vi "CMN_toMdMgr.vi"(9 "command":string) -> ()   [LabVIEW 2016]
doc: "Sends commands to the module manager"
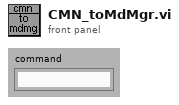
[diagram p1: front panel]
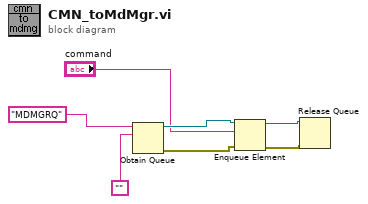
[diagram p0: block diagram]
diagram:
  n1 = Obtain Queue(name (unnamed)="MDMGRQ", element data type="") -> (queue out=w7:refnum<queue>, error out=w5:errorcluster)  [unwired: 3 in, 1 out]
  n2 = Enqueue Element(queue=w7, element="command", error in (no error)=w5) -> (queue out=w3:refnum<queue>, error out=w4:errorcluster)  [unwired: 2 out]
  n3 = Release Queue(queue=w3, error in (no error)=w4) -> ()  [unwired: 4 out]
